vi "get_frame_rate.vi"(8 "error in (no error)":errorcluster, 11 "ScanModeMG090624Camera in":refnum<class "ImagingModeMG090624Camera.lvclass">) -> (0 "error out":errorcluster, 2 "frame rate":dbl[unit], 3 "ScanModeMG090624Camera out":refnum<class "ImagingModeMG090624Camera.lvclass">)   [LabVIEW 2010, in "ImagingModeMG090624Camera.lvclass"]
uses:
  ImagingModeMG090624Camera.lvclass
  ImagingModeMG090624Camera.lvclass/ImagingModeMG090624Camera.ctl
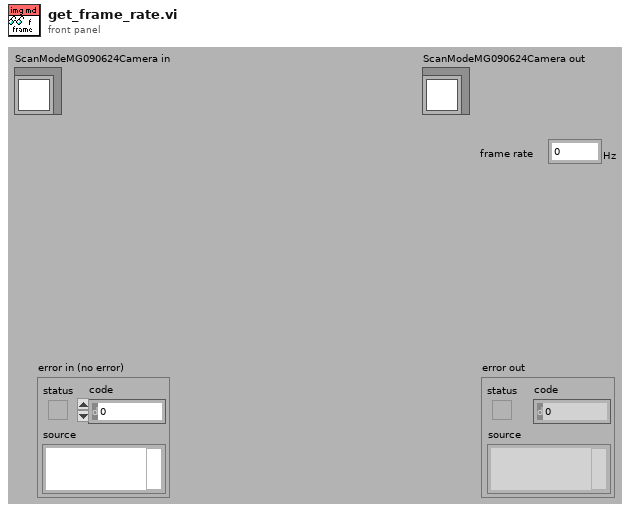
[diagram p1: front panel]
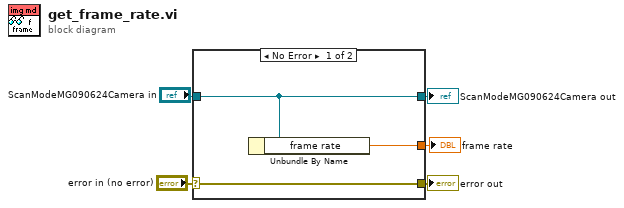
[diagram p0: block diagram]
diagram:
  n1 = case shown="No Error" "error in (no error)" {
    selector: "error in (no error)" -> [w8 w9]
    tunnel: [w8 w9] -> w4
    tunnel: [w7 w10] -> w2
    tunnel: "ScanModeMG090624Camera in" -> [w7 w10]
    tunnel: [w6 _] -> w3
    frame No Error {
      n2 = Unbundle By Name(w7) -> ("frame rate"=w6:dbl[unit])
    }
    frame Error {
    }
  }
  "error out" <- w4
  "frame rate" <- w3
  "ScanModeMG090624Camera out" <- w2
